vi "Initialize Hardware.vi"(8 "error in":errorcluster) -> (0 "error out":errorcluster)   [LabVIEW 2015]
uses:
  CAN Communication/Gas/Typedefs/Valves.ctl
  CAN Communication/Gas/Gas.lvclass
panel:
  in  "Valves":T1=33 items=["GV1"=33, "GV2"=34, "GV3"=35, "GV4"=36, "GV5"=37, "GV6"=38, "GV7"=39, "GV8"=40, "GV9"=41, "GV10"=42, "GV11"=43, "LV3"=51, "LV4"=52]
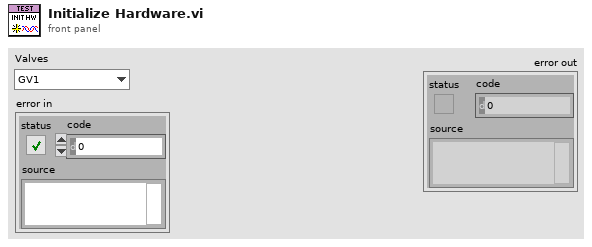
[diagram p1: front panel]
types:
  T1 = typedef "Gas.lvclass/Valves.ctl" = u16
  T2 = typedef "LVStringsAndValuesArrayTypeDef_U16.ctl" = cluster{"String":string, "Value":u16}[]
  T3 = typedef "Gas.lvclass/Session Handle.ctl" = refnum<data-value>
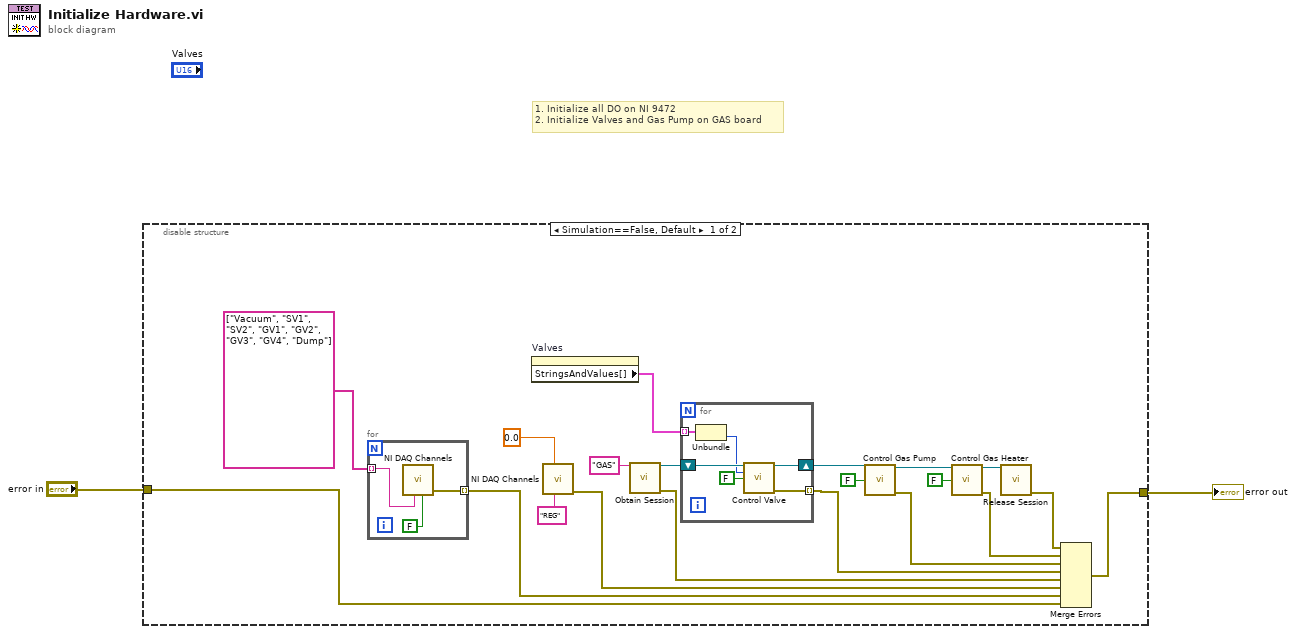
[diagram p0: block diagram]
diagram:
  # "1. Initialize all DO on NI 9472\n2. Initialize Valves and Gas Pump on GAS board"
  n1 = disable-structure shown="Simulation==False, Default" {
    disable-tunnel: "error in" -> [w12 w32]
    disable-tunnel: [w11 w32] -> w1
    frame condition #0 (active) {
      n2 = for {
        tunnel: [w31] -> w13 mode=indexing
        tunnel: string[] ["Vacuum", "SV1", "SV2", "GV1", "GV2", "GV3", "GV4", "Dump"] -> [w30] mode=indexing
        n3 = call "NI DAQ Channels.vi"("Control"=FALSE ("data"), "Channel"=w30) -> ("error out"=w31:errorcluster)  [unwired: 8 in, 1 out]
      }
      n4 = property on="Valves" class="Ring (strict)"() -> ("StringsAndValues[]"=w20:T2)  [unwired: 2 in, 2 out]
      n5 = call "NI DAQ Channels.vi"("Channel"="REG", "AO Data"=0.0 ("data")) -> ("error out"=w7:errorcluster)  [unwired: 8 in, 1 out]
      n6 = call "Obtain Session.vi"("Session  Name ()"="GAS") -> ("Session Handle"=w21:T3, "error out"=w14:errorcluster)  [unwired: 13 in]
      n7 = for {
        shift-right: [w27] -> w19
        shift-left: w21 -> [w28]
        tunnel: w20 -> [w26] mode=indexing
        tunnel: [w23] -> w15 mode=indexing
        n8 = Unbundle(w26) -> ("Value"=w25:u16)  [unwired: 1 out]
        n9 = call "Control Valve.vi"("Session Handle in"=w28, "Valves"=w25, "Energize?"=FALSE) -> ("Session Handle out"=w27:T3, "error out"=w23:errorcluster)  [unwired: 10 in, 1 out]
      }
      n10 = call "Control Gas Pump.vi"("Session Handle in"=w19, "On?"=FALSE) -> ("Session Handle out"=w5:T3, "error out"=w16:errorcluster)  [unwired: 11 in, 1 out]
      n11 = call "Control Gas Heater.vi"("Session Handle in"=w5, "On?"=FALSE) -> ("Session Handle out"=w4:T3, "error out"=w3:errorcluster)  [unwired: 11 in, 1 out]
      n12 = call "Release Session.vi"("Session Handle"=w4) -> ("error out"=w17:errorcluster)  [unwired: 14 in]
      n13 = Merge Errors(w17, w3, w16, w15, w14, w7, w13, w12) -> (w11:errorcluster)
    }
    frame condition #1 {
    }
  }
  "error out" <- w1
